vi "GT Pvt Table Ex.vi"(0 "cardNum":i16, 1 "pPos":dbl, 2 "pVelEnd":dbl, 5 "tableId":i16, 7 "count":i32, 9 "pTime":dbl, 11 "error in (no error)":errorcluster caption="错误输入（无错误）", 12 "pVelBegin":dbl) -> (3 "pPos out":dbl, 4 "pVelEnd out":dbl, 6 "function return":i16, 10 "pTime out":dbl, 14 "pVelBegin out":dbl, 15 "error out":errorcluster caption="错误输出")   [LabVIEW 2014, in "gts.lvlib"]
doc: "GT_API GT_PvtTableEx(short cardNum,short tableId,long count,double *pTime,double *pPos,double *pVelBegin,double *pVelEnd);"
uses:
  gts.lvlib
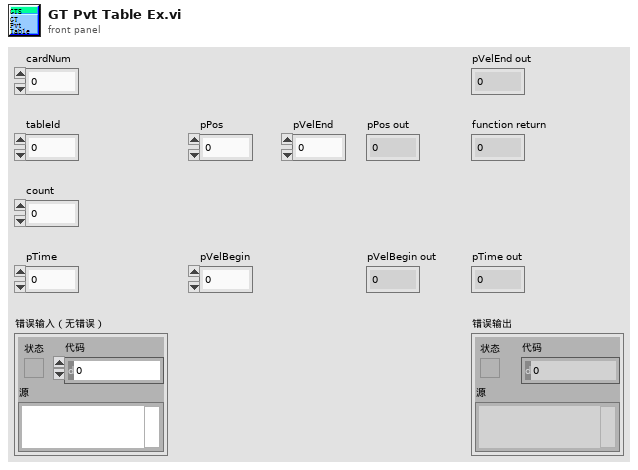
[diagram p1: front panel]
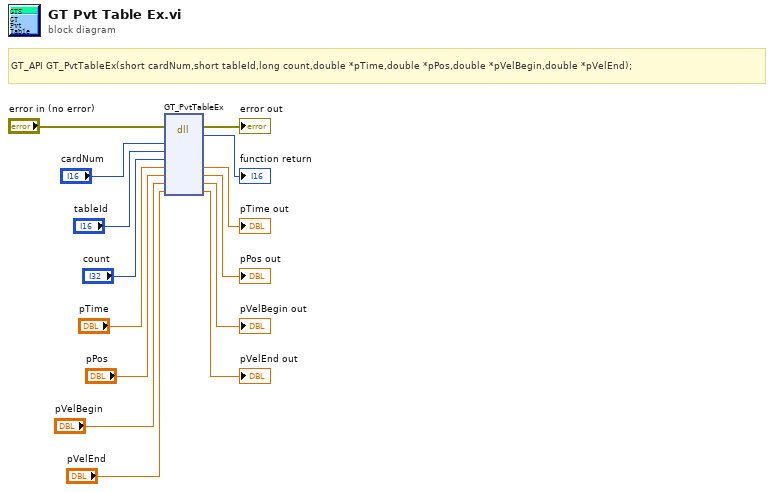
[diagram p0: block diagram]
diagram:
  # "GT_API GT_PvtTableEx(short cardNum,short tableId,long count,double *pTime,double *pPos,double *pVelBegin,double *pVelEnd);"
  n1 = dll-call lib="PTH2habs D固高科技资料GTS控制卡GTS卡18年上半年资料dllVC32bit\nmulti_cardgts.*" fn="GT_PvtTableEx"(error in="error in (no error)", "cardNum"="cardNum", "tableId"="tableId", "count"="count", "pTime"="pTime", "pPos"="pPos", "pVelBegin"="pVelBegin", "pVelEnd"="pVelEnd") -> (error out=→"error out":errorcluster, →"function return":i16, "pTime"=→"pTime out":dbl, "pPos"=→"pPos out":dbl, "pVelBegin"=→"pVelBegin out":dbl, "pVelEnd"=→"pVelEnd out":dbl)  [unwired: 5 in, 1 out]
